vi "Discover.vi"(8 "error in (no error)":errorcluster, 9 "Timeout (ms)":i32=2000, 10 "Port":i32=58431) -> (0 "error out":errorcluster, 3 "Discovered Devices":T1[](array[typedef]))   [LabVIEW 2021, in "BS120x Driver.lvlib"]
uses:
  BS120x Driver.lvlib
  DiscoveredDevice.ctl
  TypeDefs/UnitType.ctl
  TypeDefs/Protocol.ctl
  d267861c-3c49-4d0f-b8fe-a75797aacc06.vi
  BS120x.lvclass
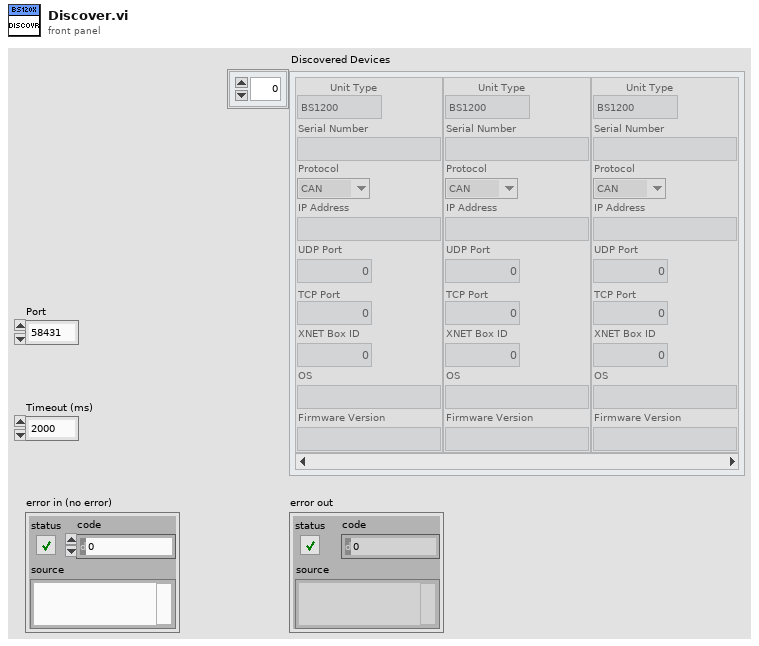
[diagram p1: front panel]
types:
  T1 = typedef "BS120x Driver.lvlib/DiscoveredDevice.ctl" = cluster{"Unit Type":T2, "Serial Number":string, "Protocol":T3, "IP Address":string, "UDP Port":u16, "TCP Port":u16, "XNET Box ID":u8, "OS":string, "Firmware Version":string}
  T2 = typedef "BS120x Driver.lvlib/BS120x.lvclass/UnitType.ctl" = enum16{"BS1200", "BS1201"}
  T3 = typedef "BS120x Driver.lvlib/BS120x.lvclass/Protocol.ctl" = enum16{"CAN", "Ethernet"}
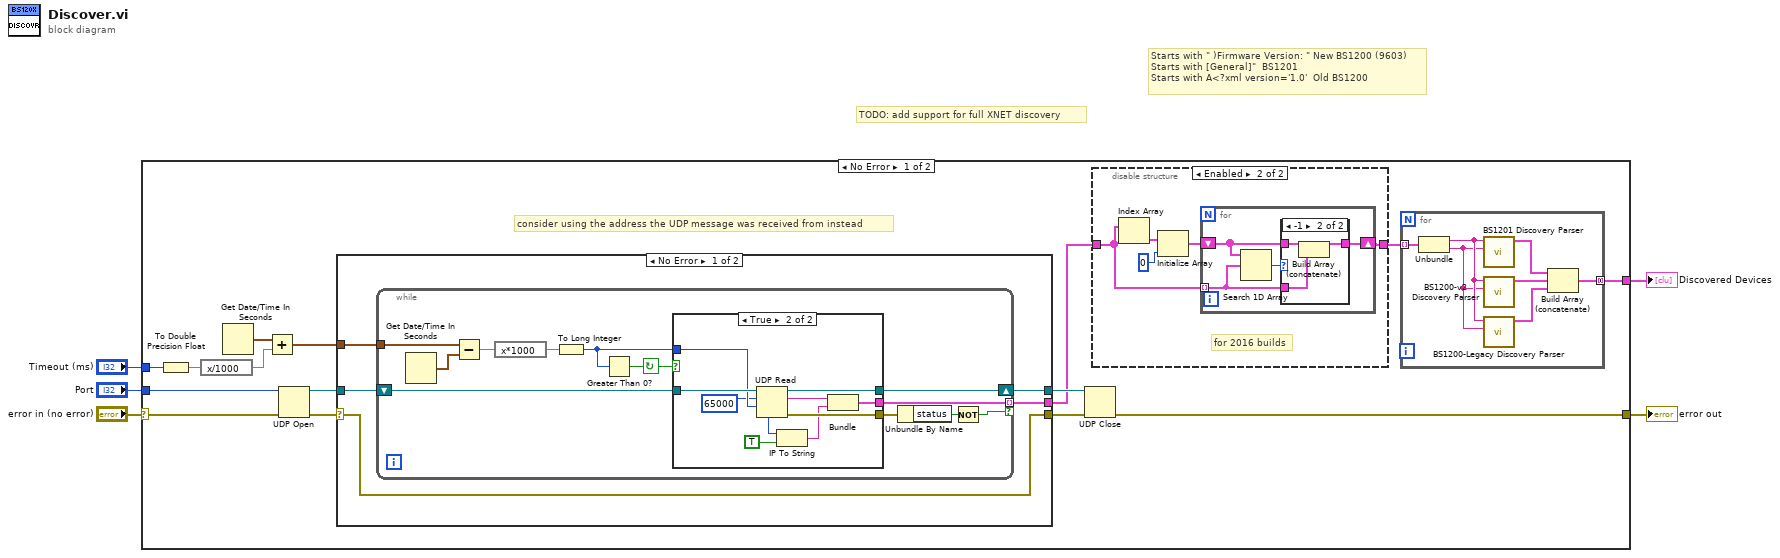
[diagram p0: block diagram]
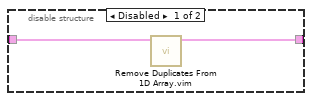
[diagram p2: hidden frame]
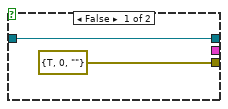
[diagram p4: hidden frame]
diagram:
  # "Starts with \" )Firmware Version: \" New BS1200 (9603)\nStarts with [General]\"  BS1201\nStarts with A<?xml version='1.0'  Old BS1200"
  # "TODO: add support for full XNET discovery"
  n1 = case shown="No Error" "error in (no error)" {
    selector: "error in (no error)" -> [w14 w74]
    tunnel: "Timeout (ms)" -> [w18 _]
    tunnel: "Port" -> [w12 _]
    tunnel: [w8 w74] -> w2
    tunnel: [w7 _] -> w1
    frame No Error {
      # "consider using the address the UDP message was received from instead"
      n2 = To Double Precision Float(number=w18) -> (double precision float=w17:dbl)
      n3 = expression code="x/1000"(w17) -> (w16:dbl)
      n4 = Get Date/Time In Seconds() -> (seconds since 1Jan1904=w19:timestamp)
      n5 = Add(x=w19, y=w16) -> (x+y=w15:timestamp)
      n6 = UDP Open(8:w14, 11:w12) -> (port=w11:refnum<k16>, 0:w13:errorcluster)  [unwired: 3 in, 1 out]
      n7 = case shown="No Error" w13 {
        selector: w13 -> [w45 w73]
        tunnel: [w45 w73] -> w20
        tunnel: w15 -> [w47 _]
        tunnel: w11 -> [w46 w72]
        tunnel: [w44 w72] -> w10
        tunnel: [w43 _] -> w9
        frame No Error {
          n8 = while {
            tunnel: w47 -> [w57]
            tunnel: [w53] -> w43 mode=indexing if=w48
            shift-right: [w49] -> w44
            shift-left: w46 -> [w59]
            stop <- w52 continue-if-true
            n9 = Get Date/Time In Seconds() -> (seconds since 1Jan1904=w58:timestamp)
            n10 = Subtract(x=w57, y=w58) -> (x-y=w56:dbl)
            n11 = expression code="x*1000"(w56) -> (w55:dbl)
            n12 = To Long Integer(number=w55) -> (32bit integer=w54:i32)
            n13 = Greater Than 0?(x=w54) -> (x > 0?=w52:bool)
            n14 = case shown="True" w52 {
              tunnel: w59 -> [w60 w71]
              tunnel: w54 -> [_ w70]
              tunnel: [_ w63] -> w53
              tunnel: [errorcluster {"status"=TRUE, "code"=0, "source"=""} ("error out") w68] -> w51
              tunnel: [w60 w67] -> w49
              frame False {
              }
              frame True {
                n15 = UDP Read(connection ID=w71, max size (548)=65000, timeout ms (25000)=w70) -> (data out=w69:string, error out=w68:errorcluster, 3:w67:refnum<k16>, 6:w65:u32)  [unwired: 1 in, 1 out]
                n16 = IP To String(1:TRUE ("dot notation? (F)"), 2:w65) -> (0:w62:string)
                n17 = Bundle("data out"=w69, "name"=w62) -> (w63:cluster{"data out":string, "name":string})  [unwired: 1 in]
              }
            }
            n18 = Unbundle By Name(w51) -> ("status"=w50:bool)
            n19 = Not(x=w50) -> (.not. x?=w48:bool)
          }
        }
        frame Error {
        }
      }
      n20 = UDP Close(connection ID=w10, 8:w20) -> (error out=w8:errorcluster)  [unwired: 1 out]
      n21 = disable-structure shown="Enabled" {
        disable-tunnel: w9 -> [w22 w24]
        disable-tunnel: [w21 w23] -> w6
        frame Disabled {
          n22 = call "Remove Duplicates From 1D Array.vim"("array"=w22) -> ("array with duplicates removed"=w21:cluster{"data out":string, "name":string}[])  [unwired: 10 in]
        }
        frame Enabled {
          # "for 2016 builds"
          n23 = Index Array(array=w24) -> (element=w25:cluster{"data out":string, "name":string})  [unwired: 1 in]
          n24 = Initialize Array(w25, 0 ("Dimension Size")) -> (w26:cluster{"data out":string, "name":string}[])
          n25 = for {
            tunnel: w24 -> [w30] mode=indexing
            shift-right: [w29] -> w23
            shift-left: w26 -> [w28]
            n26 = Search 1D Array(1D array=w28, element=w30) -> (index of element=w31:i32)  [unwired: 1 in]
            n27 = case shown="-1" w31 {
              tunnel: w30 -> [_ w35]
              tunnel: [w32 w33] -> w29
              tunnel: w28 -> [w32 w34]
              frame Default {
              }
              frame -1 {
                n28 = Build Array (concatenate)(w34, w35) -> (w33:cluster{"data out":string, "name":string}[])
              }
            }
          }
        }
      }
      n29 = for {
        tunnel: w6 -> [w38] mode=indexing
        tunnel: [w42] -> w7 mode=concatenating
        n30 = Unbundle(w38) -> ("data out"=w37:string, "name"=w36:string)
        n31 = call "BS1201 Discovery Parser.vi"("IP Address"=w36, "Discovery String"=w37) -> ("Devices"=w40:T1[])  [unwired: 9 in]
        n32 = call "BS1200-v2 Discovery Parser.vi"("IP Address"=w36, "Discovery String"=w37) -> ("Devices"=w41:T1[])  [unwired: 9 in]
        n33 = call "BS1200-Legacy Discovery Parser.vi"("IP Address"=w36, "Discovery String"=w37) -> ("Devices"=w39:T1[])  [unwired: 9 in]
        n34 = Build Array (concatenate)(w40, w41, w39) -> (w42:T1[])
      }
    }
    frame Error {
    }
  }
  "Discovered Devices" <- w1
  "error out" <- w2
